vi "SDCP SMF Transmitter and Receiver - Live Plot - Obtain Instantaeneous Data Points.vi"(0 "Raw frame":T2, 2 "Initialize ?":bool, 3 "error in (no error)":errorcluster) -> (5 "Instantaeneous data":T1(array[cluster]), 7 "error out":errorcluster)   [LabVIEW 2020]
uses:
  Typedefs/SDCP - Standard Message Frame Parameters - FGV - commands.ctl
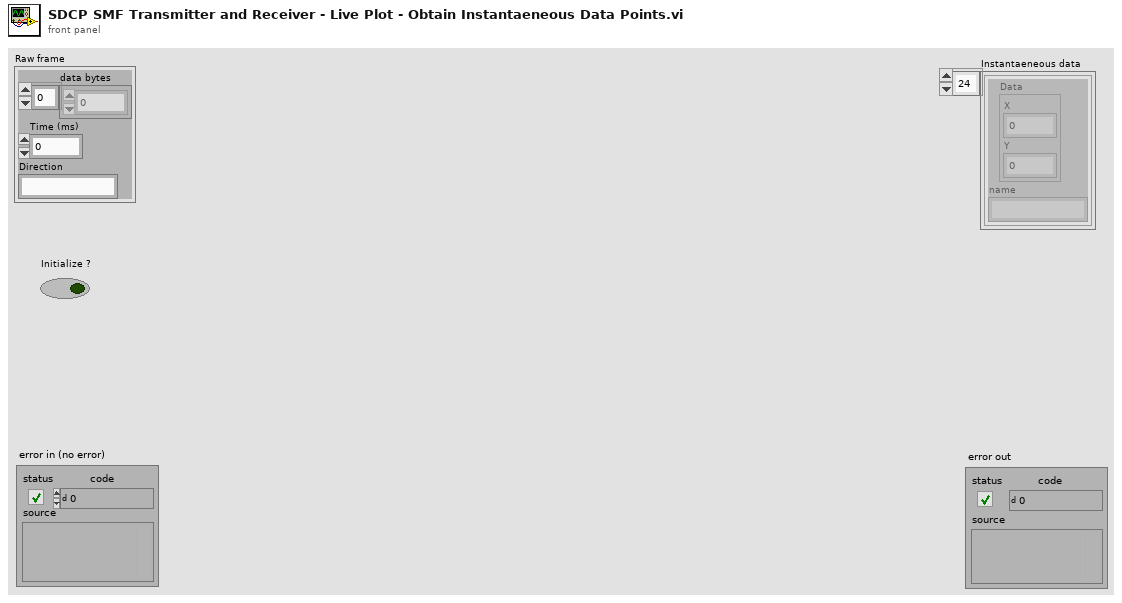
[diagram p1: front panel]
types:
  T1 = cluster{"Data":cluster{"X":dbl, "Y":dbl}, "name":string}[]
  T2 = cluster{"data bytes":u8[], "Time (ms)":u32, "Direction":string}
  T3 = typedef "SDCP - Standard Message Frame Parameters - FGV - commands.ctl" = enum16{"Write descriptors", "Read descriptors", "Read values", "Load parameters from file", "Write values", "Read all descriptors"}
  T4 = cluster{"Data":cluster{"X":dbl, "Y":dbl}, "name":string}
  T5 = typedef "SDCP - SMF parameter descriptors.ctl" = cluster{"Frame name":string, "Frame ID":i32, "Data type":string, "Start Position":i32, "Length":i32, "Factor":dbl, "Offset":dbl, "Parameter name":string, "Value":string}
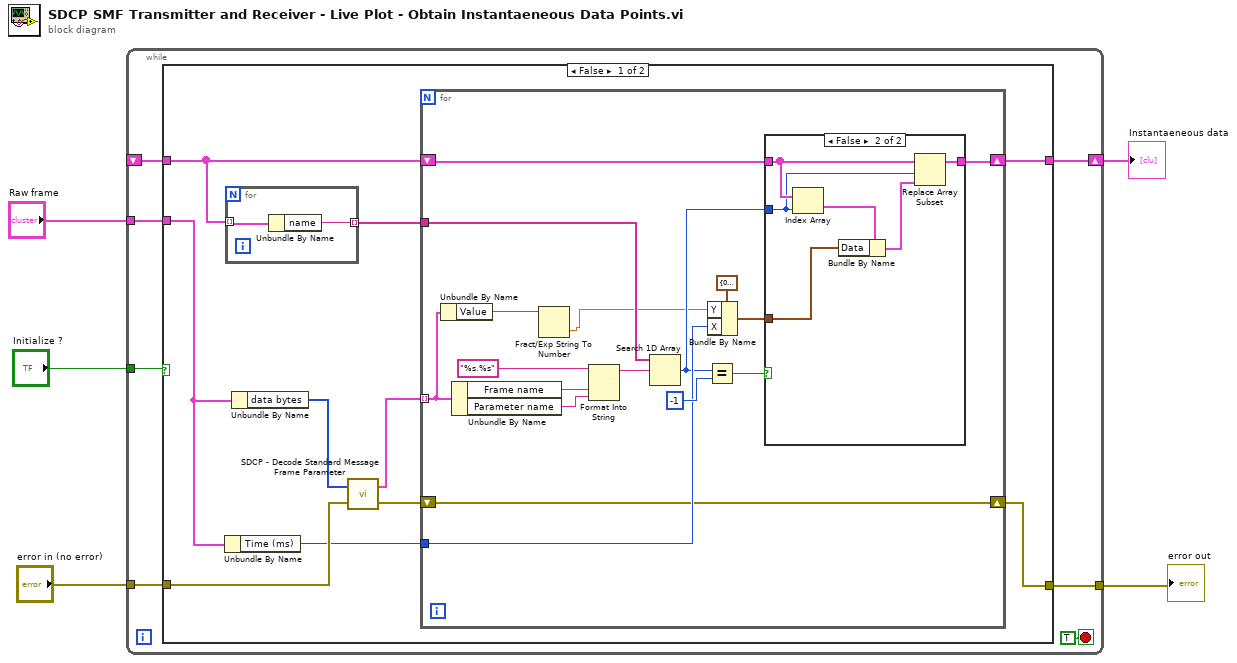
[diagram p0: block diagram]
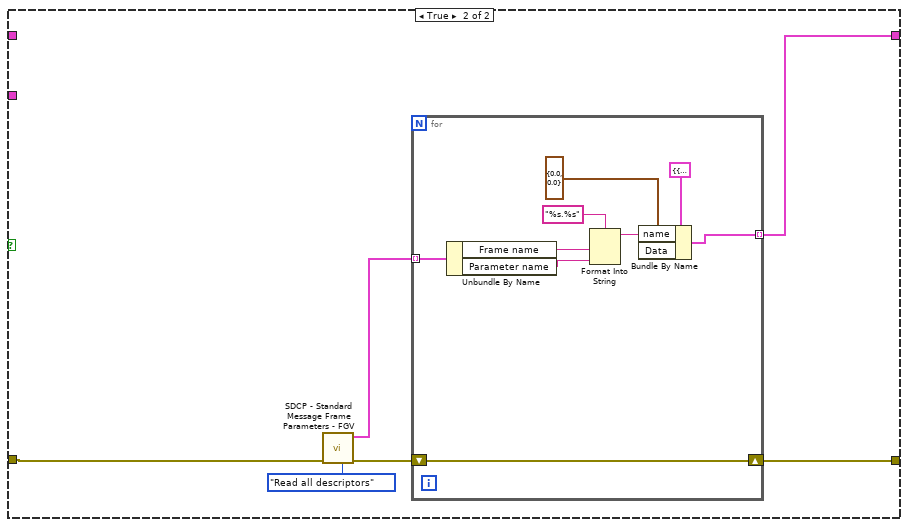
[diagram p3: hidden frame]
diagram:
  n1 = while {
    tunnel: "error in (no error)" -> [w10]
    tunnel: "Initialize ?" -> [w11]
    shift-right: [w8] -> w1
    shift-left: _ -> [w7]
    tunnel: [w9] -> w3
    tunnel: "Raw frame" -> [w6]
    stop <- TRUE stop-if-true
    n2 = case shown="False" w11 {
      tunnel: w10 -> [w21 w54]
      tunnel: [w13 w50] -> w9
      tunnel: [w20 w49] -> w8
      tunnel: w7 -> [w17 _]
      tunnel: w6 -> [w15 _]
      frame False {
        n3 = Unbundle By Name(w15) -> ("Time (ms)"=w14:u32)
        n4 = for {
          tunnel: w17 -> [w24] mode=indexing
          tunnel: [w23] -> w16 mode=indexing
          n5 = Unbundle By Name(w24) -> ("name"=w23:string)
        }
        n6 = Unbundle By Name(w15) -> ("data bytes"=w22:u8[])
        n7 = call "SDCP - Decode Standard Message Frame Parameter.vi"("error in (no error)"=w21, "Bytes in"=w22) -> ("error out"=w19:errorcluster, "SMF Parameters out"=w18:T5[])
        n8 = for {
          shift-right: [w34] -> w20
          shift-left: w17 -> [w35]
          tunnel: w18 -> [w37] mode=indexing
          tunnel: w16 -> [w38]
          tunnel: w14 -> [w29]
          shift-right: [w27] -> w13
          shift-left: w19 -> [w27]
          n9 = Unbundle By Name(w37) -> ("Value"=w36:string)
          n10 = Unbundle By Name(w37) -> ("Frame name"=w41:string, "Parameter name"=w40:string)
          n11 = Fract/Exp String To Number(string=w36) -> (number=w25:dbl)  [unwired: 3 in, 1 out]
          n12 = Format Into String(format string="%s.%s", w41, w40) -> (resulting string=w32:string)  [unwired: 2 in, 1 out]
          n13 = Search 1D Array(1D array=w38, element=w32) -> (index of element=w26:i32)  [unwired: 1 in]
          n14 = Equal?(x=w26, y=-1) -> (x = y?=w30:bool)
          n15 = Bundle By Name(cluster=cluster{"X":dbl, "Y":dbl} {"X"=0.0, "Y"=0.0} ("Data"), "Y"=w25, "X"=w29) -> (w28:cluster{"X":dbl, "Y":dbl})
          n16 = case shown="False" w30 {
            tunnel: w35 -> [w42 w47]
            tunnel: [w42 w48] -> w34
            tunnel: w26 -> [_ w43]
            tunnel: w28 -> [_ w45]
            frame True {
            }
            frame False {
              n17 = Index Array(array=w47, index=w43) -> (element=w46:T4)
              n18 = Bundle By Name(cluster=w46, "Data"=w45) -> (w44:T4)
              n19 = Replace Array Subset(array=w47, new element=w44, index=w43) -> (w48:T1)
            }
          }
        }
      }
      frame True {
        n20 = call "SDCP - Standard Message Frame Parameters - FGV.vi"("error in (no error)"=w54, "Command"=SDCP_-_Standard_Message_Frame_Parameters_-_FGV_-_commands."Read all descriptors") -> ("SMF Parameters descriptors out"=w52:T5[], "error out"=w51:errorcluster)  [unwired: 5 in]
        n21 = for {
          tunnel: w52 -> [w63] mode=indexing
          shift-right: [w57] -> w50
          shift-left: w51 -> [w57]
          tunnel: [w56] -> w49 mode=indexing
          n22 = Unbundle By Name(w63) -> ("Frame name"=w60:string, "Parameter name"=w59:string)
          n23 = Format Into String(format string="%s.%s", w60, w59) -> (resulting string=w58:string)  [unwired: 2 in, 1 out]
          n24 = Bundle By Name(cluster=T4 {"Data"={"X"=0.0, "Y"=0.0}, "name"=""}, "name"=w58, "Data"=cluster{"X":dbl, "Y":dbl} {"X"=0.0, "Y"=0.0}) -> (w56:T4)
        }
      }
    }
  }
  "error out" <- w3
  "Instantaeneous data" <- w1
